vi "Voronoi_Triangle Center.vi"(9 "Y":dbl[](array[numeric]), 10 "X":dbl[](array[numeric]), 11 "Triangle":i32[](array[numeric])) -> (3 "Delaunay Center":dbl[](array[numeric]) format="%.2f")   [LabVIEW 2017, in "NI_AAL_Geometry.lvlib"]
uses:
  <vilib>/Analysis/NI_AAL_Geometry.lvlib
  <vilib>/Analysis/7linalg.llb/Solve Linear Equations (single right hand).vi
  <vilib>/Analysis/baseanly.llb/Solve Linear Equations By Cholesky.vi
  <vilib>/Analysis/baseanly.llb/Real Matrix to Compact Array.vi
  <vilib>/Analysis/baseanly.llb/Real Compact Tri-Matrix Linear Eqs.vi
  <vilib>/Analysis/7linalg.llb/Solve Linear Eqs (General).vi
  <vilib>/Analysis/7linalg.llb/Solve Linear Eqs (Gen, single right hand).vi
  <vilib>/Analysis/NI_AALPro.lvlib
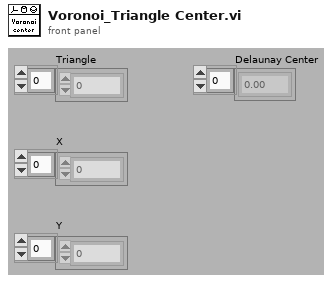
[diagram p1: front panel]
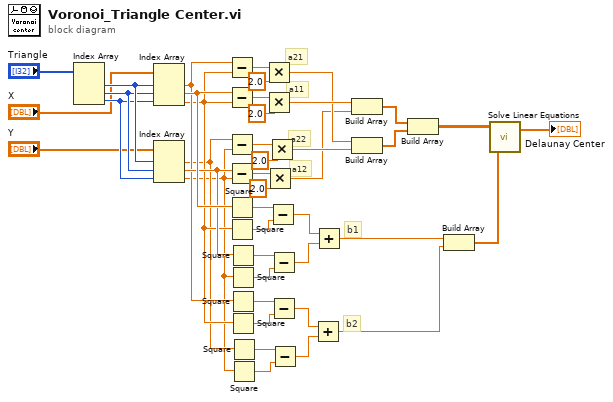
[diagram p0: block diagram]
diagram:
  # "b2"
  # "b1"
  # "a22"
  # "a21"
  # "a12"
  # "a11"
  n1 = Index Array(array="Triangle") -> (element #1=w43:i32, element #2=w42:i32, element #3=w41:i32)  [unwired: 3 in]
  n2 = Index Array(array="X", index #1=w43, index #2=w42, index #3=w41) -> (element #1=w14:dbl, element #2=w24:dbl, element #3=w13:dbl)
  n3 = Index Array(array="Y", index #1=w43, index #2=w42, index #3=w41) -> (element #1=w12:dbl, element #2=w19:dbl, element #3=w11:dbl)
  n4 = Subtract(x=w14, y=w13) -> (x-y=w33:dbl)
  n5 = Subtract(x=w24, y=w13) -> (x-y=w36:dbl)
  n6 = Subtract(x=w12, y=w11) -> (x-y=w29:dbl)
  n7 = Subtract(x=w19, y=w11) -> (x-y=w31:dbl)
  n8 = Square(x=w24) -> (x^2=w23:dbl)
  n9 = Square(x=w13) -> (x^2=w22:dbl)
  n10 = Square(x=w19) -> (x^2=w21:dbl)
  n11 = Square(x=w11) -> (x^2=w20:dbl)
  n12 = Square(x=w14) -> (x^2=w18:dbl)
  n13 = Square(x=w13) -> (x^2=w17:dbl)
  n14 = Square(x=w12) -> (x^2=w16:dbl)
  n15 = Square(x=w11) -> (x^2=w15:dbl)
  n16 = Multiply(x=w33, y=2.0) -> (x*y=w27:dbl)
  n17 = Multiply(x=w36, y=2.0) -> (x*y=w28:dbl)
  n18 = Multiply(x=w31, y=2.0) -> (x*y=w25:dbl)
  n19 = Multiply(x=w29, y=2.0) -> (x*y=w26:dbl)
  n20 = Subtract(x=w23, y=w22) -> (x-y=w10:dbl)
  n21 = Subtract(x=w21, y=w20) -> (x-y=w9:dbl)
  n22 = Subtract(x=w18, y=w17) -> (x-y=w8:dbl)
  n23 = Subtract(x=w16, y=w15) -> (x-y=w7:dbl)
  n24 = Add(x=w8, y=w7) -> (x+y=w5:dbl)
  n25 = Add(x=w10, y=w9) -> (x+y=w6:dbl)
  n26 = Build Array(w28, w25) -> (w40:dbl[])
  n27 = Build Array(w27, w26) -> (w39:dbl[])
  n28 = Build Array(w40, w39) -> (w37:dbl[][])
  n29 = Build Array(w6, w5) -> (w38:dbl[])
  n30 = call-poly <vilib>:"Solve Linear Equations.vi"("Known Vector"=w38, "Input Matrix"=w37) -> ("Solution Vector"=→"Delaunay Center":dbl[])  [unwired: 1 in, 1 out]
